vi "Sweep WL ISPP.vi"(8 "error in (no error)":errorcluster, 9 "Sweep outfile":path, 10 "addr":i32, 11 "instrument handle":refnum<k15>) -> (0 "error out":errorcluster, 1 "final current (A)":dbl, 2 "final resistance (ohm)":dbl, 3 "instrument handle out":refnum<k15>)   [LabVIEW 2018]
uses:
  <vilib>/Utility/file.llb/Write Delimited Spreadsheet (DBL).vi
panel:
  out "i":i32
  out "PW":i32
  out "BL voltage (V)":dbl
  out "WL voltage (V)":dbl
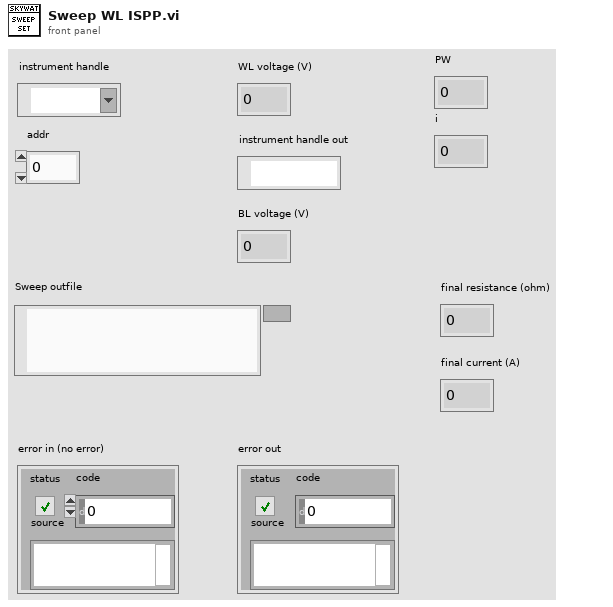
[diagram p1: front panel]
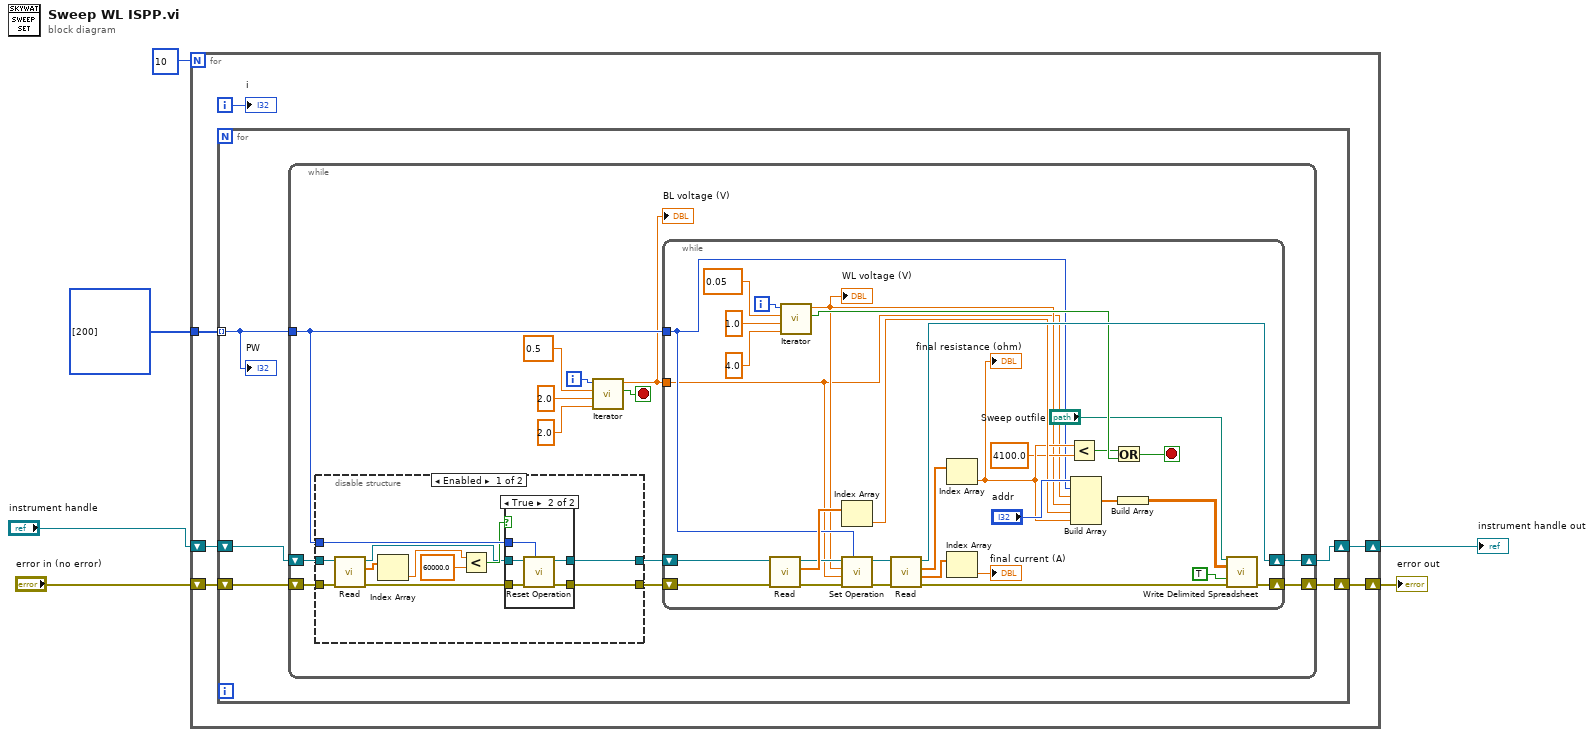
[diagram p0: block diagram]
diagram:
  n1 = for {
    N: 10 -> [_]
    tunnel: i32[] [200] -> [w8]
    shift-right: [w12] -> w6
    shift-left: "instrument handle" -> [w11]
    shift-right: [w9] -> w3
    shift-left: "error in (no error)" -> [w10]
    i -> [w7]
    n2 = for {
      shift-right: [w17] -> w12
      shift-left: w11 -> [w16]
      shift-right: [w14] -> w9
      shift-left: w10 -> [w15]
      tunnel: w8 -> [w13] mode=indexing
      n3 = while {
        shift-right: [w27] -> w17
        shift-left: w16 -> [w21]
        shift-right: [w26] -> w14
        shift-left: w15 -> [w20]
        tunnel: w13 -> [w24]
        i -> [w28]
        stop <- w23 stop-if-true
        n4 = disable-structure shown="Enabled" {
          disable-tunnel: w24 -> [w41 _]
          disable-tunnel: w21 -> [w40 w50]
          disable-tunnel: w20 -> [w39 w49]
          disable-tunnel: [w38 w50] -> w19
          disable-tunnel: [w37 w49] -> w18
          frame Enabled {
            n5 = call "Read.vi"("error in (no error)"=w39, "instrument handle"=w40) -> ("error out"=w32:errorcluster, "resistances (ohm)"=w36:dbl[], "instrument handle out"=w33:refnum<k15>)  [unwired: 6 in, 1 out]
            n6 = Index Array(array=w36) -> (element=w31:dbl)  [unwired: 1 in]
            n7 = Less?(x=w31, y=60000.0) -> (x < y?=w34:bool)
            n8 = case shown="True" w34 {
              tunnel: w33 -> [w43 w48]
              tunnel: w32 -> [w42 w47]
              tunnel: [w43 w46] -> w38
              tunnel: [w42 w45] -> w37
              tunnel: w41 -> [_ w44]
              frame False {
              }
              frame True {
                n9 = call "Reset Operation.vi"("PW"=w44, "error in (no error)"=w47, "instrument handle"=w48) -> ("error out"=w45:errorcluster, "instrument handle out"=w46:refnum<k15>)  [unwired: 7 in]
              }
            }
          }
          frame Disabled {
          }
        }
        n10 = call "Iterator.vi"("Final Value"=2.0 ("y"), "Initial Value"=2.0 ("y"), "Step"=0.5 ("x"), "i"=w28) -> ("End Loop"=w23:bool, "Current Value"=w22:dbl)  [unwired: 6 in]
        "BL voltage (V)" <- w22
        n11 = while {
          shift-right: [w71] -> w27
          shift-left: w19 -> [w52]
          shift-right: [w74] -> w26
          shift-left: w18 -> [w51]
          tunnel: w22 -> [w53]
          tunnel: w24 -> [w56]
          i -> [w81]
          stop <- w65 stop-if-true
          n12 = call "Read.vi"("error in (no error)"=w51, "instrument handle"=w52) -> ("error out"=w59:errorcluster, "resistances (ohm)"=w67:dbl[], "instrument handle out"=w60:refnum<k15>)  [unwired: 6 in, 1 out]
          n13 = call "Iterator.vi"("Final Value"=4.0 ("y"), "Initial Value"=1.0 ("y"), "Step"=0.05 ("x"), "i"=w81) -> ("End Loop"=w64:bool, "Current Value"=w54:dbl)  [unwired: 6 in]
          "WL voltage (V)" <- w54
          n14 = Index Array(array=w67) -> (element=w66:dbl)  [unwired: 1 in]
          n15 = call "Set Operation.vi"("PW"=w56, "error in (no error)"=w59, "BLV"=w53, "WLV"=w54, "instrument handle"=w60) -> ("error out"=w58:errorcluster, "instrument handle out"=w57:refnum<k15>)  [unwired: 5 in]
          n16 = call "Read.vi"("error in (no error)"=w58, "instrument handle"=w57) -> ("error out"=w72:errorcluster, "currents (A)"=w69:dbl[], "resistances (ohm)"=w70:dbl[], "instrument handle out"=w71:refnum<k15>)  [unwired: 6 in]
          n17 = Index Array(array=w70) -> (element=w63:dbl)  [unwired: 1 in]
          "final resistance (ohm)" <- w63
          n18 = Index Array(array=w69) -> (element=→"final current (A)":dbl)  [unwired: 1 in]
          n19 = Less?(x=w63, y=4100.0 ("x")) -> (x < y?=w61:bool)
          n20 = Build Array("addr", w56, w53, w54, w66, w63) -> (w76:dbl[])
          n21 = Or(x=w61, y=w64) -> (x .or. y?=w65:bool)
          n22 = Build Array(w76) -> (w77:dbl[][])
          n23 = call-poly <vilib>:"Write Delimited Spreadsheet.vi"("file path (dialog if empty)"="Sweep outfile", "2D data"=w77, "append to file? (new file:F)"=TRUE, "error in (no error)"=w72) -> ("error out"=w74:errorcluster)  [unwired: 10 in, 1 out]
        }
      }
      "PW" <- w13
    }
    "i" <- w7
  }
  "error out" <- w3
  "instrument handle out" <- w6
